vi "Mode of String Array.vi"(8 "error in":errorcluster, 11 "Input Elements":string[](array[string])=["apple", "apple", "kiwi", "orange", "apple", "orange"]) -> (0 "error out":errorcluster, 2 "most frequent Count":i32, 3 "most frequent":string)   [LabVIEW 2018]
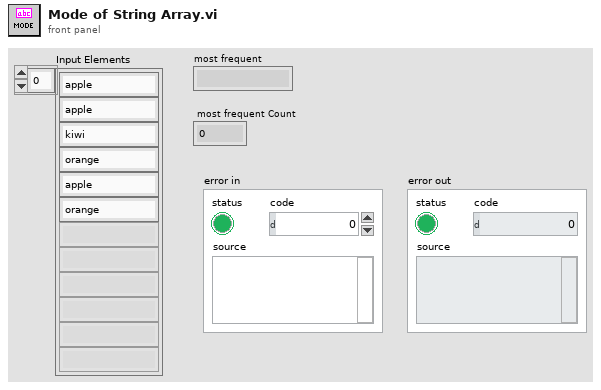
[diagram p1: front panel]
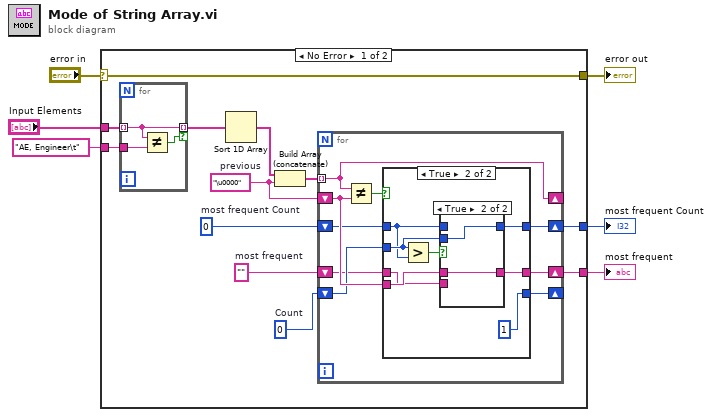
[diagram p0: block diagram]
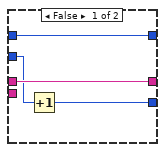
[diagram p2: hidden frame]
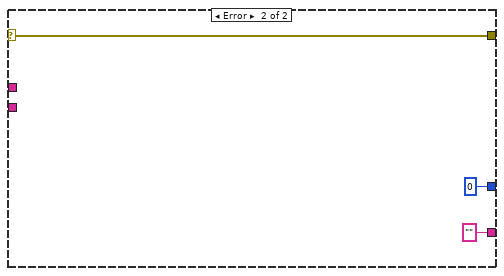
[diagram p4: hidden frame]
diagram:
  n1 = case shown="No Error" "error in" {
    selector: "error in" -> [w7 w49]
    tunnel: [w12 "" ("most frequent")] -> w6
    tunnel: [w11 0 ("most frequent Count")] -> w5
    tunnel: "Input Elements" -> [w10 _]
    tunnel: "AE, Engineer\t" ("t") -> [w9 _]
    tunnel: [w7 w49] -> w1
    frame No Error {
      w15 = 0  # most frequent Count
      w16 = ""  # most frequent
      w17 = 0  # Count
      w13 = "\u0000"  # previous
      n2 = for {
        tunnel: w10 -> [w20] mode=indexing
        tunnel: w9 -> [w21]
        tunnel: [w20] -> w8 mode=indexing if=w19
        n3 = Not Equal?(x=w20, y=w21) -> (x != y?=w19:bool)
      }
      n4 = Sort 1D Array(array=w8) -> (sorted array=w18:string[])
      n5 = Build Array (concatenate)(w18, w13) -> (w14:string[])
      n6 = for {
        tunnel: w14 -> [w30] mode=indexing
        shift-right: [w30] -> _
        shift-left: w13 -> [w27]
        shift-right: [w26] -> _
        shift-left: w17 -> [w25]
        shift-right: [w28] -> w12
        shift-left: w16 -> [w24]
        shift-right: [w22] -> w11
        shift-left: w15 -> [w23]
        n7 = Not Equal?(x=w30, y=w27) -> (x != y?=w29:bool)
        n8 = case shown="True" w29 {
          tunnel: [w34 w39] -> w28
          tunnel: w27 -> [_ w38]
          tunnel: [w31 1] -> w26
          tunnel: w25 -> [w32 w40]
          tunnel: w24 -> [w34 w37]
          tunnel: [w33 w41] -> w22
          tunnel: w23 -> [w33 w36]
          frame False {
            n9 = Increment(x=w32) -> (x+1=w31:i32)
          }
          frame True {
            n10 = Greater?(x=w40, y=w36) -> (0:w42:bool)
            n11 = case shown="True" w42 {
              tunnel: [w43 w46] -> w41
              tunnel: w40 -> [_ w46]
              tunnel: [w44 w45] -> w39
              tunnel: w38 -> [_ w45]
              tunnel: w37 -> [w44 _]
              tunnel: w36 -> [w43 _]
              frame False {
              }
              frame True {
              }
            }
          }
        }
      }
    }
    frame Error {
    }
  }
  "error out" <- w1
  "most frequent" <- w6
  "most frequent Count" <- w5
